vi "Struct (Single Type).vi"(6 "Typedef name":string, 7 "Typedef struct? (F)":bool, 8 "Struct name":string, 9 "Data type":string="double", 10 "Variable names":string[](array[string]), 11 "String in":string) -> (3 "String out":string)   [LabVIEW 2014, in "C Header Generator.lvlib"]
uses:
  C Header Generator.lvlib
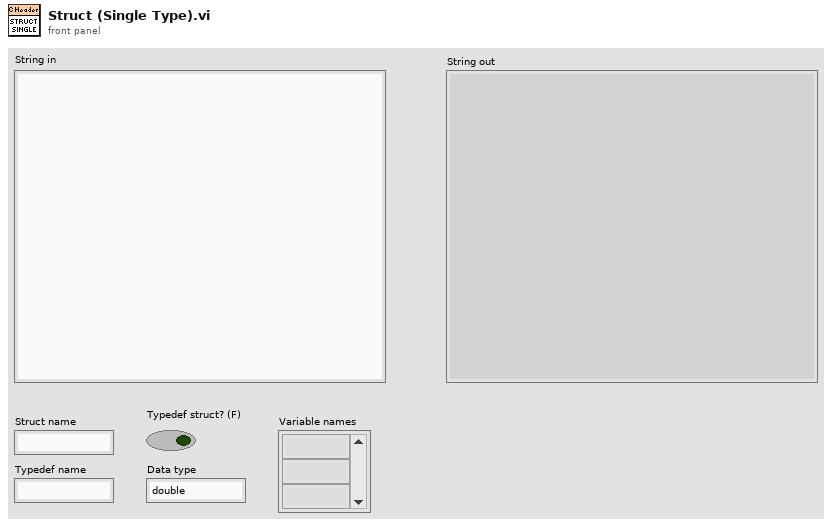
[diagram p1: front panel]
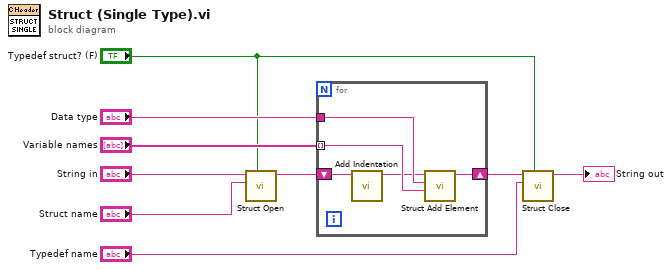
[diagram p0: block diagram]
diagram:
  n1 = call "Struct Open.vi"("Typedef struct? (F)"="Typedef struct? (F)", "Struct name"="Struct name", "String in"="String in") -> ("String out"=w5:string)  [unwired: 8 in]
  n2 = for {
    shift-right: [w14] -> w9
    shift-left: w5 -> [w11]
    tunnel: "Data type" -> [w13]
    tunnel: "Variable names" -> [w12] mode=indexing
    n3 = call "Add Indentation.vi"("String in"=w11) -> ("String out"=w10:string)  [unwired: 10 in]
    n4 = call "Struct Add Element.vi"("Element name"=w12, "Element type"=w13, "String in"=w10) -> ("String out"=w14:string)  [unwired: 8 in]
  }
  n5 = call "Struct Close.vi"("Typedef struct? (F)"="Typedef struct? (F)", "Typedef name"="Typedef name", "String in"=w9) -> ("String out"=→"String out":string)  [unwired: 8 in]
